vi "test Reading an Already Read Result Gets The Same Result.vi"(8 "error in (no error)":errorcluster, 11 "TestCase in":refnum<class "Task Tests.lvclass">) -> (0 "error out":errorcluster, 3 "TestCase out":refnum<class "Task Tests.lvclass">)   [LabVIEW 2017, in "Task Tests.lvclass"]
uses:
  Task Tests.lvclass
  <vilib>/addons/_JKI Toolkits/VI Tester/TestCase.llb/TestCase.lvclass
  Futures/Task/Task.lvclass
  C:/Program Files (x86)/National Instruments/LabVIEW 2017/vi.lib/addons/_JKI Toolkits/VI Tester/TestCase.llb/TestCase.lvclass
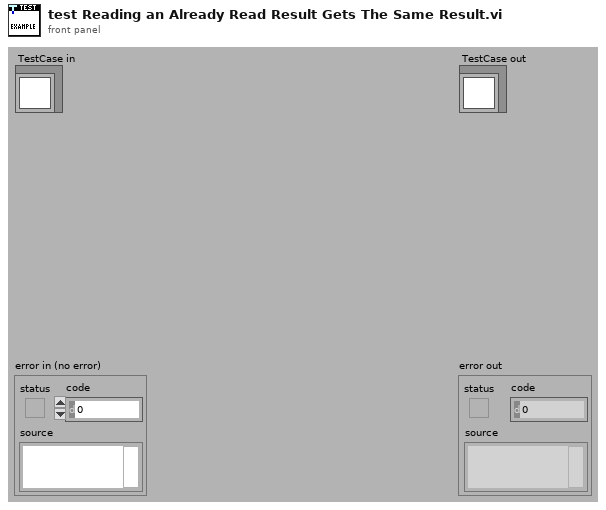
[diagram p1: front panel]
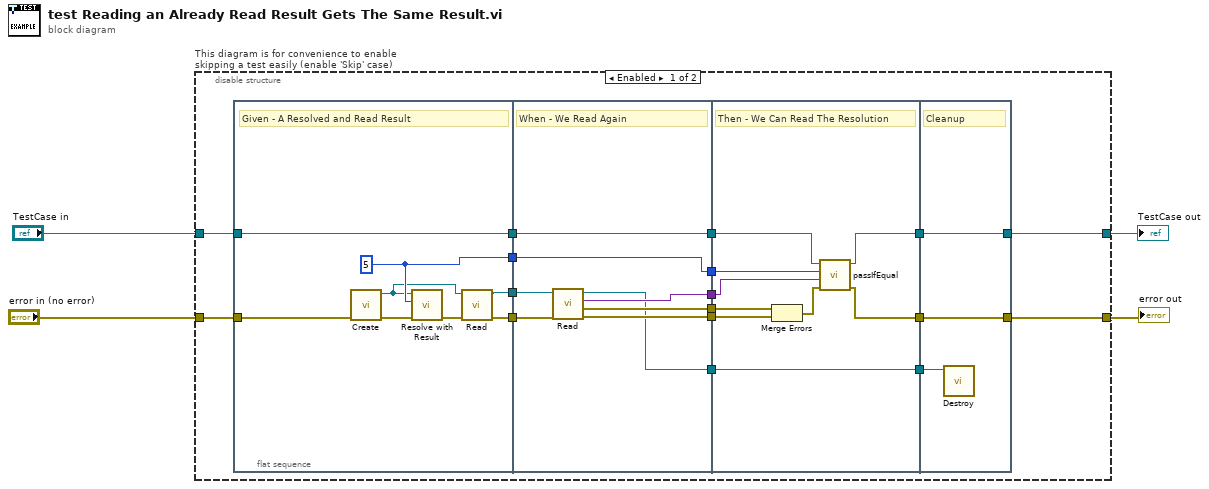
[diagram p0: block diagram]
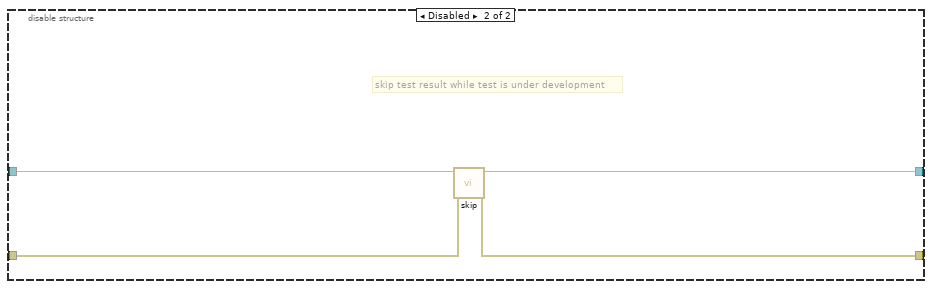
[diagram p2: hidden frame]
diagram:
  n1 = disable-structure "This diagram is for convenience to enable skipping a test easily (enable 'Skip' case)" shown="Enabled" {
    disable-tunnel: "TestCase in" -> [w17 w53]
    disable-tunnel: [w15 w51] -> w1
    disable-tunnel: [w14 w52] -> w3
    disable-tunnel: "error in (no error)" -> [w16 w50]
    frame Enabled {
      n2 = flat-sequence {
        tunnel: w16 -> [w28]
        tunnel: w17 -> [w29]
        tunnel: [w29] -> w21
        tunnel: [w26] -> w12
        tunnel: [w24] -> w8
        tunnel: [w22] -> w7
        tunnel: [w37] -> w20
        tunnel: w21 -> [w37]
        tunnel: [w36] -> w13
        tunnel: w12 -> [w36]
        tunnel: [w35] -> w11
        tunnel: [w34] -> w10
        tunnel: [w33] -> w9
        tunnel: w8 -> [w32]
        tunnel: w7 -> [w31]
        tunnel: [w30] -> w6
        tunnel: [w45] -> w19
        tunnel: [w44] -> w18
        tunnel: w20 -> [w46]
        tunnel: w13 -> [w42]
        tunnel: w11 -> [w41]
        tunnel: w10 -> [w40]
        tunnel: w9 -> [w39]
        tunnel: w6 -> [w38]
        tunnel: [w38] -> w5
        tunnel: [w48] -> w14
        tunnel: [w49] -> w15
        tunnel: w19 -> [w49]
        tunnel: w18 -> [w48]
        tunnel: w5 -> [w47]
        frame #0 {
          w26 = 5
          # "Given - A Resolved and Read Result"
          n3 = call "Create.vi"("error in (no error)"=w28) -> ("error out"=w27:errorcluster, "Result out"=w23:refnum<class "Task.lvclass">)  [unwired: 9 in]
          n4 = call "Resolve with Result.vi"("error in (no error)"=w27, "Result"=w26, "Result in"=w23) -> ("error out"=w25:errorcluster)  [unwired: 8 in]
          n5 = call "Read.vi"("error in (no error)"=w25, "Result in"=w23) -> ("error out"=w24:errorcluster, "Result Out"=w22:refnum<class "Task.lvclass">)  [unwired: 5 in, 3 out]
        }
        frame #1 {
          # "When - We Read Again"
          n6 = call "Read.vi"("error in (no error)"=w32, "Result in"=w31) -> ("error out"=w35:errorcluster, "result error"=w34:errorcluster, "Result value"=w33:variant, "Result Out"=w30:refnum<class "Task.lvclass">)  [unwired: 5 in, 1 out]
        }
        frame #2 {
          # "Then - We Can Read The Resolution"
          n7 = Merge Errors(w40, w41) -> (w43:errorcluster)
          n8 = call-dynamic "passIfEqual.vi"("error in (no error)"=w43, "y"=w39, "x"=w42, "TestCase in"=w46) -> ("error out"=w44:errorcluster, "TestCase out"=w45:refnum<class "Task Tests.lvclass">)  [unwired: 6 in]
        }
        frame #3 {
          # "Cleanup"
          n9 = call "Destroy.vi"("Result in"=w47) -> ()  [unwired: 10 in, 1 out]
        }
      }
    }
    frame Disabled {
      # "skip test result while test is under development"
      n10 = call <vilib>:"skip.vi"("error in (no error)"=w50, "TestCase in"=w53) -> ("error out"=w52:errorcluster, "TestCase out"=w51:refnum<class "Task Tests.lvclass">)  [unwired: 8 in]
    }
  }
  "error out" <- w3
  "TestCase out" <- w1
